vi "Read Parent Attributes.vi"(7 "Actor in":refnum<class "Actor.lvclass">) -> (2 "Parent Attributes":refnum<data-value>)   [LabVIEW 2020, in "jettl.lvlib" / "Actor Specific.lvlib"]
uses:
  Actor Specific.lvlib
  Actor/Actor.lvclass
  Msg/Msg.lvclass
  Transport/Transport.lvclass
  Attributes Metadata/Attributes Metadata.lvclass
  Msgs.ctl
  jettl.lvlib
  Attributes.ctl
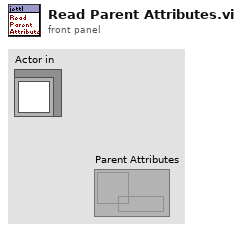
[diagram p1: front panel]
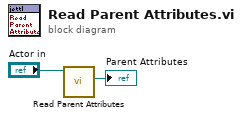
[diagram p0: block diagram]
diagram:
  n1 = call-dynamic "Read Parent Attributes.vi"("Actor in"="Actor in") -> ("Parent Attributes"=→"Parent Attributes":refnum<data-value>)  [unwired: 10 in]
